vi "Pockels modulation-Gen AO seq for non-funct img.vi"(9 "Imaging Protocol":T1, 11 "Setup/Logging queue element":T2={"Imaging Protocol"=enum."Live Imaging", "Number of Trials"=0, "Frame Size"=512, "# Averaged frames"=0, "Dwell time (us)"=0.0, "Index of Z-plane"=0, "Timelapse?"=FALSE, "Logging process is active"=FALSE, "Speed logging enabled"=FALSE, "tdms file ref"=refnum, "path"=path "", "Trial Number"=0, "Expected # points acquired"=FALSE, "Manually stopped"=FALSE, "Last trial"=FALSE, "Ch0 data"=[], "Ch1 data"=[], "Ref Data"=[], "Ref Frame Time"=[], "Image Time"=[], "Continuous Time"=[], "Ref X Length"=0, "Ref Y Length"=0, "# Ref Averaged frames"=0, "Ref Dwell time (us)"=0.0, "Points acquired"={"Ch0 last trial"=0, "Ch1 last trial"=0, "All trials"=0}, "HW Timings File"=refnum} {"Ref Dwell time (us)" format="%#.6g"; "Frame Size" items=["100X100"=100, "128X128"=128, "200X200"=200, "256X256"=256, "512X512"=512, "1024x1024"=1024, "2048x2048"=2048]; "Dwell time (us)" format="%#.6g"}) -> (1 "Pockels modulation AO sequence":dbl[](array[numeric]), 2 "Sampling period (us)":dbl format="%#_6f", 3 "Length of sequence (ms)":dbl format="%#_6f", 4 "Data length (points)":i32)   [LabVIEW 2020]
uses:
  Typedefs/Logging queue element.ctl
  Typedefs/Imaging Protocols enum.ctl
  Typedefs/Frame Size.ctl
  Typedefs/Acquired points count.ctl
  Typedefs/Pockels mod gen variables cluster.ctl
  Typedefs/Pockels modulation Internal cluster 1.ctl
  Typedefs/Rounding type.ctl
  Global Variables/General Globals.vi
  Globals/gl_Pockels control globals.vi
panel:
  out "Pockels modulation waveform":dbl[](graph)
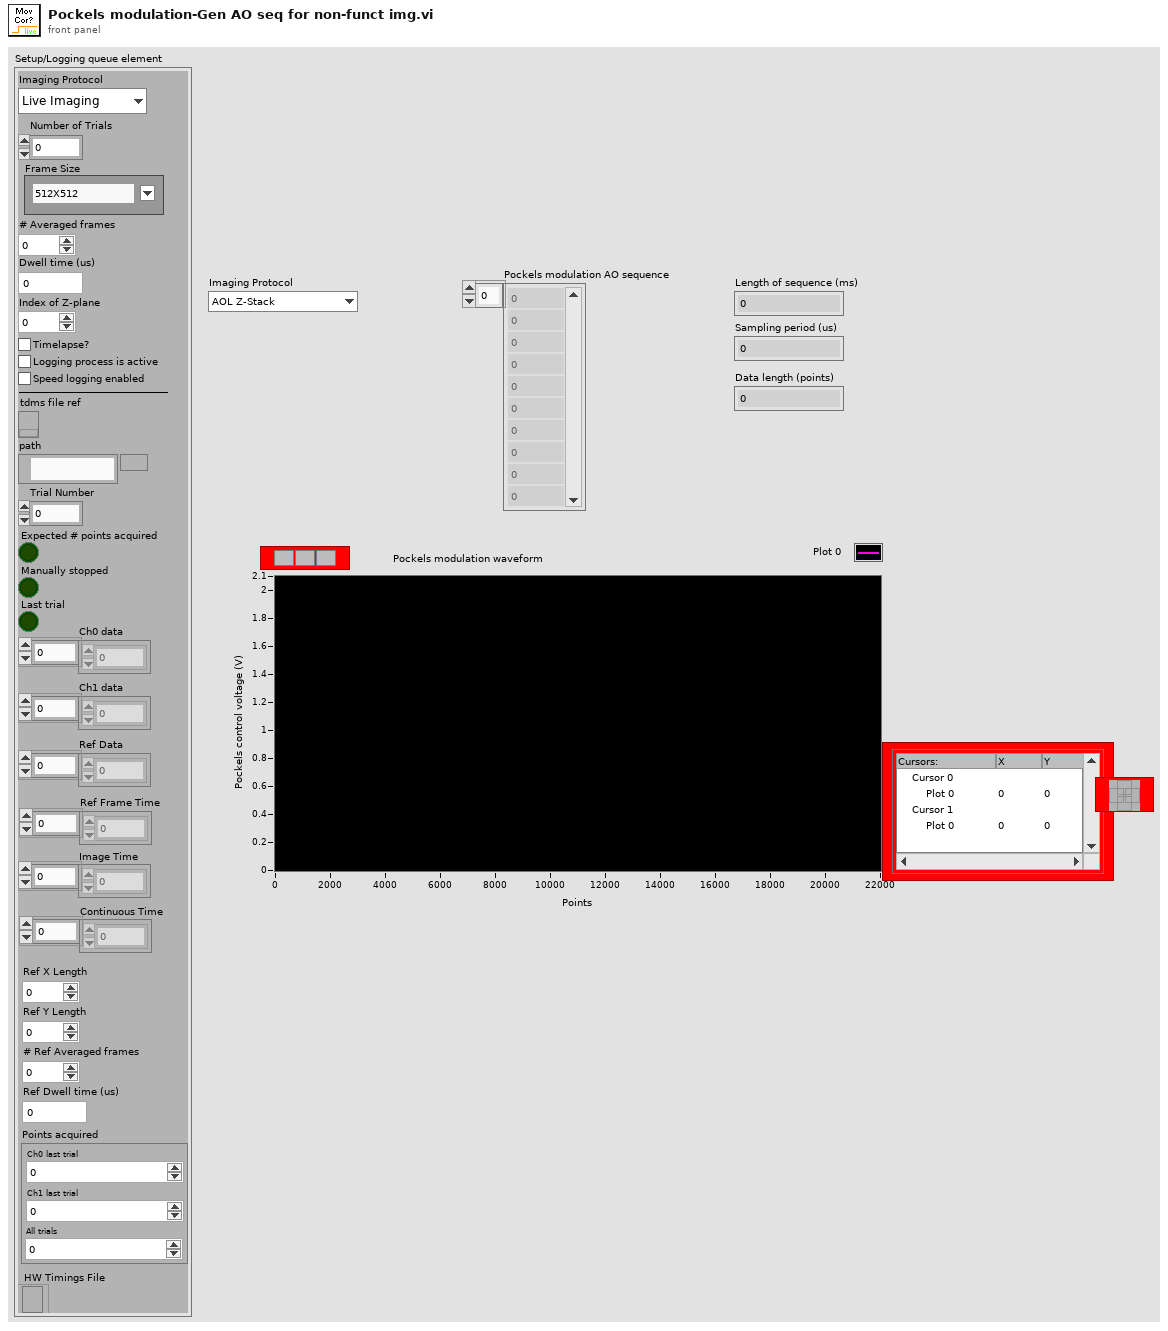
[diagram p1: front panel]
types:
  T1 = typedef "Imaging Protocols enum.ctl" = enum16{"AOL Z-Stack", "Motor Z Stack", "Functional Acquisition", "Single Plane Acquisition", "Volume Acquisition", "Live Imaging", "Live Plane Imaging", "Live Volume Imaging"}
  T2 = typedef "Logging queue element.ctl" = cluster{"Imaging Protocol":T1, "Number of Trials":u16, "Frame Size":T3, "# Averaged frames":u16, "Dwell time (us)":dbl, "Index of Z-plane":i32, "Timelapse?":bool, "Logging process is active":bool, "Speed logging enabled":bool, "tdms file ref":refnum<k34>, "path":path, "Trial Number":i32, "Expected # points acquired":bool, "Manually stopped":bool, "Last trial":bool, "Ch0 data":u32[], "Ch1 data":u32[], "Ref Data":u32[], "Ref Frame Time":u64[], "Image Time":u64[], "Continuous Time":u64[], "Ref X Length":u16, "Ref Y Length":u16, "# Ref Averaged frames":u16, "Ref Dwell time (us)":dbl, "Points acquired":T4, "HW Timings File":refnum<file>}
  T3 = typedef "Frame Size.ctl" = u16
  T4 = typedef "Acquired points count.ctl" = cluster{"Ch0 last trial":u64, "Ch1 last trial":u64, "All trials":u64}
  T5 = typedef "Pockels modulation Internal cluster 1.ctl" = cluster{"Pockels ON \"Pre\" (samples)":i32, "Direction (+-Inf)":T6, "Additional duration to stay ON (samples)":i32, "Not the last ROI":bool}
  T6 = typedef "Rounding type.ctl" = enum16{"No rounding", "Toward +Inf", "Toward -Inf"}
  T7 = typedef "Pockels mod gen variables cluster.ctl" = cluster{"Dwell time":dbl, "Number of frame lines":i32, "Number of points in a line":i32, "Index of Z-plane":i32, "Pockels \"Low\" time (us)":dbl, "Sample Clock Rate":dbl, "Imaging Protocol":T1}
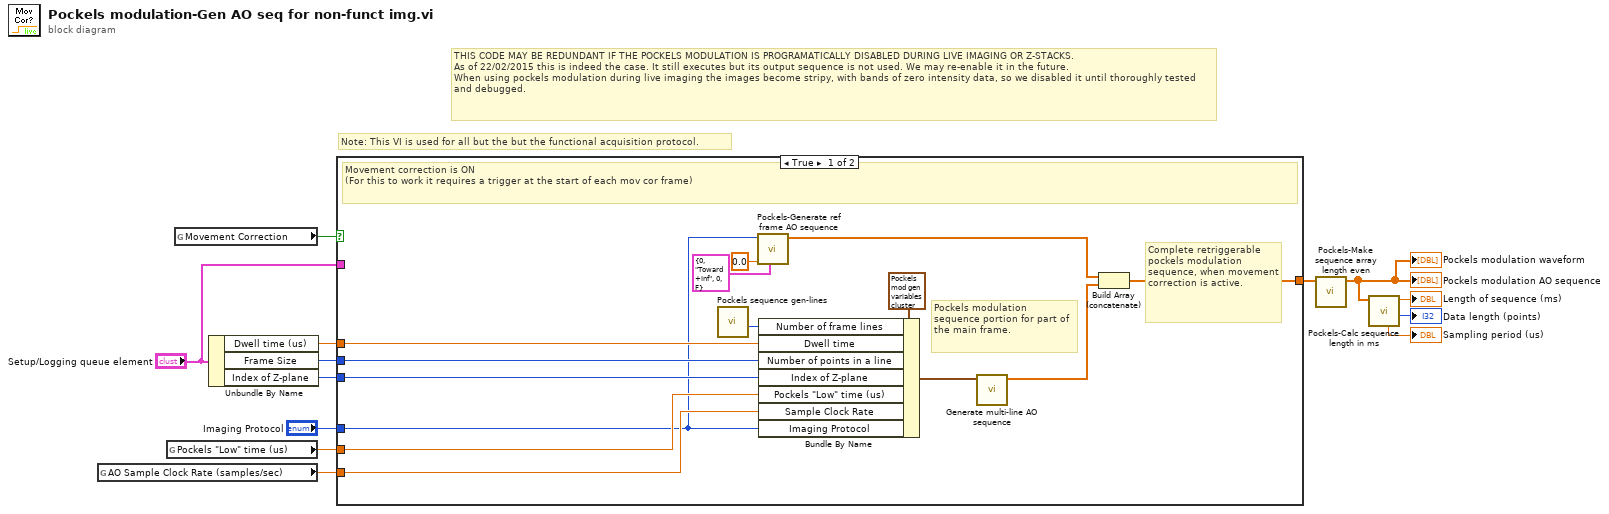
[diagram p0: block diagram]
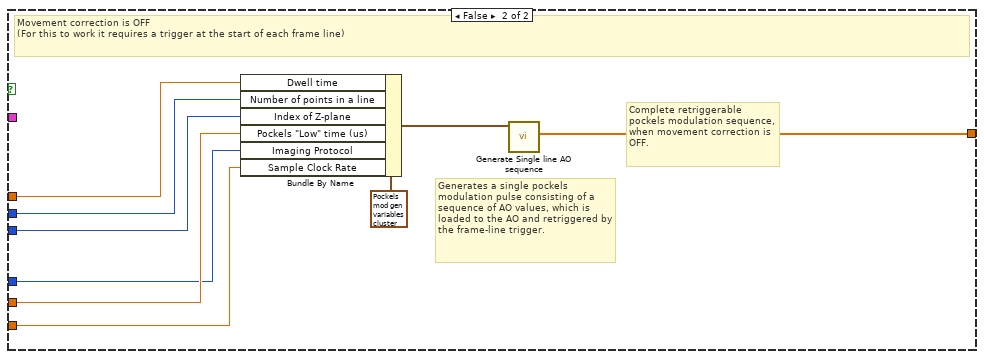
[diagram p2: hidden frame]
diagram:
  # "THIS CODE MAY BE REDUNDANT IF THE POCKELS MODULATION IS PROGRAMATICALLY DISABLED DURING LIVE IMAGING OR Z-STACKS.\nAs of 22/02/2015 this is indeed the case. It still executes but its output sequence is not used. We may re-enable it in the future.\nWhen using pockels modulation during live imaging the images become stripy, with bands of zero intensity data, so we disabled it until thoroughly tested and debugged."
  # "Note: This VI is used for all but the but the functional acquisition protocol."
  n1 = global read "General Globals.vi" "AO Sample Clock Rate (samples/sec)"() -> (w5:dbl)
  n2 = global read "gl_Pockels control globals.vi" "Pockels \"Low\" time (us)"() -> (w8:dbl)
  n3 = global read "General Globals.vi" "Movement Correction"() -> (w9:bool)
  n4 = Unbundle By Name("Setup/Logging queue element") -> ("Dwell time (us)"=w10:dbl, "Frame Size"=w11:T3, "Index of Z-plane"=w12:i32)
  n5 = case shown="True" w9 {
    tunnel: w10 -> [w23 w33]
    tunnel: w11 -> [w27 w32]
    tunnel: [w20 w36] -> w6
    tunnel: w12 -> [w26 w31]
    tunnel: "Imaging Protocol" -> [w16 w29]
    tunnel: w8 -> [w24 w30]
    tunnel: w5 -> [w18 w28]
    tunnel: "Setup/Logging queue element" -> [_ _]
    frame True {
      # "Complete retriggerable pockels modulation sequence, when movement correction is active."
      # "Pockels modulation sequence portion for part of the main frame."
      # "Movement correction is ON\n(For this to work it requires a trigger at the start of each mov cor frame)"
      n6 = call "Pockels sequence gen-lines.vi"() -> ("Lines in chunk for the trigger period target (ms)"=w19:i32)  [unwired: 9 in, 2 out]
      n7 = call "Pockels-Generate ref frame AO sequence.vi"("Cluster"=T5 {"Pockels ON \"Pre\" (samples)"=0, "Direction (+-Inf)"=enum."Toward +Inf", "Additional duration to stay ON (samples)"=0, "Not the last ROI"=FALSE}, "Previous excess us (us)"=0.0, "Imaging Protocol"=w16) -> ("Pockels modulation sequence"=w17:dbl[])  [unwired: 4 in, 4 out]
      n8 = Bundle By Name(cluster=T7 {"Dwell time"=0.0, "Number of frame lines"=512, "Number of points in a line"=0, "Index of Z-plane"=0, "Pockels \"Low\" time (us)"=0.0, "Sample Clock Rate"=0.0, "Imaging Protocol"=enum."AOL Z-Stack"} ("Variables"), "Number of frame lines"=w19, "Dwell time"=w23, "Number of points in a line"=w27, "Index of Z-plane"=w26, "Pockels \"Low\" time (us)"=w24, "Sample Clock Rate"=w18, "Imaging Protocol"=w16) -> (w22:T7)
      n9 = call "Generate multi-line AO sequence.vi"("Variables"=w22) -> ("Pockels modulation sequence"=w21:dbl[])  [unwired: 10 in]
      n10 = Build Array (concatenate)(w17, w21) -> (w20:dbl[])
    }
    frame False {
      # "Complete retriggerable pockels modulation sequence, when movement correction is OFF."
      # "Generates a single pockels modulation pulse consisting of a sequence of AO values, which is loaded to the AO and retriggered by the frame-line trigger."
      # "Movement correction is OFF\n(For this to work it requires a trigger at the start of each frame line)"
      n11 = Bundle By Name(cluster=T7 {"Dwell time"=0.0, "Number of frame lines"=512, "Number of points in a line"=0, "Index of Z-plane"=0, "Pockels \"Low\" time (us)"=0.0, "Sample Clock Rate"=0.0, "Imaging Protocol"=enum."AOL Z-Stack"} ("Variables"), "Dwell time"=w33, "Number of points in a line"=w32, "Index of Z-plane"=w31, "Pockels \"Low\" time (us)"=w30, "Imaging Protocol"=w29, "Sample Clock Rate"=w28) -> (w35:T7)
      n12 = call "Generate Single line AO sequence.vi"("Variables"=w35) -> ("Single line AO sequence"=w36:dbl[])  [unwired: 10 in]
    }
  }
  n13 = call "Pockels-Make sequence array length even.vi"("Single line AO sequence in"=w6) -> ("Single line AO sequence out"=w4:dbl[])  [unwired: 10 in]
  "Pockels modulation AO sequence" <- w4
  "Pockels modulation waveform" <- w4
  n14 = call "Pockels-Calc sequence length in ms.vi"("Pockels modulation sequence in"=w4) -> ("Sequence length (points)"=→"Data length (points)":i32, "Sequence length (ms)"=→"Length of sequence (ms)":dbl, "Sampling period (us)"=→"Sampling period (us)":dbl)  [unwired: 8 in]
